vi "A x Vector.vi"(2 "Vector":dbl[](array[numeric]) format="%.2f", 3 "A":T1) -> (0 "error":i32, 1 "A x Vector":dbl[](array[numeric]) format="%.2f")   [LabVIEW 2017, in "NI_AALBase.lvlib"]
doc: "Performs the multiplication of two input matrices or an input matrix and an input vector. The data types you wire to the <B>A</B> and <B>B</B> inputs determine the polymorphic instance to use."
uses:
  <vilib>/Analysis/NI_AALBase.lvlib
  <vilib>/Analysis/Matrix/Datatypes/RealMatrix.ctl
  <resource>/lvanlys.dll
  <vilib>/Analysis/Matrix/NI_Matrix.lvlib
panel:
  # "A x Vector"
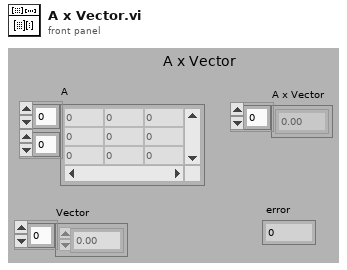
[diagram p1: front panel]
types:
  T1 = typedef "NI_Matrix.lvlib/RealMatrix.ctl" = dbl[][]
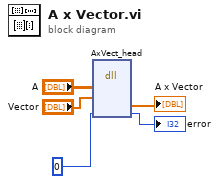
[diagram p0: block diagram]
diagram:
  n1 = dll-call lib="e:/builds/penguin/labview/branches/2017/dev/dist/resource/lvanlys.*" fn="AxVect_head"("A"="A", "Vector"="Vector", 0) -> ("A x Vector"=→"A x Vector":dbl[], →"error":i32)  [unwired: 7 in, 2 out]
